vi "例程03-For、while循环、条件结构、事件结构.vi"() -> ()   [LabVIEW 2018]
panel:
  out "数值":dbl
  in  "事件结构测试":bool
  out "while次数 2":i32
  out "布尔":bool
  out "while次数":i32
  out "波形图表 2":dbl(graph)
  out "for次数":i32
  out "波形图表":dbl(graph)
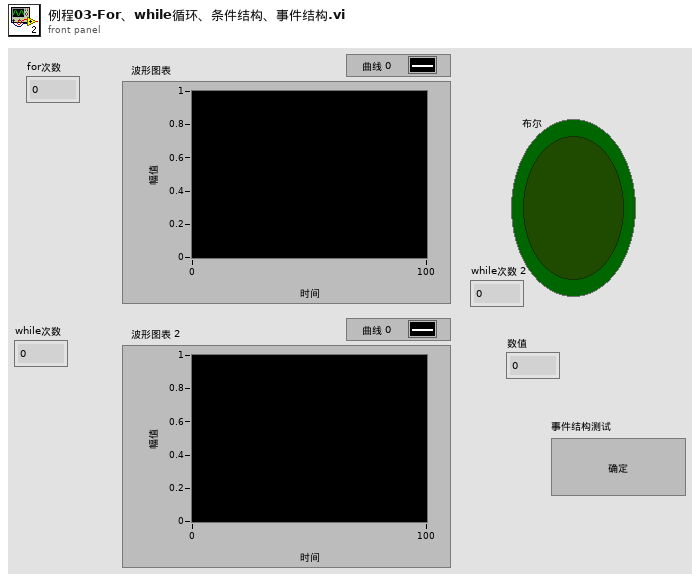
[diagram p1: front panel]
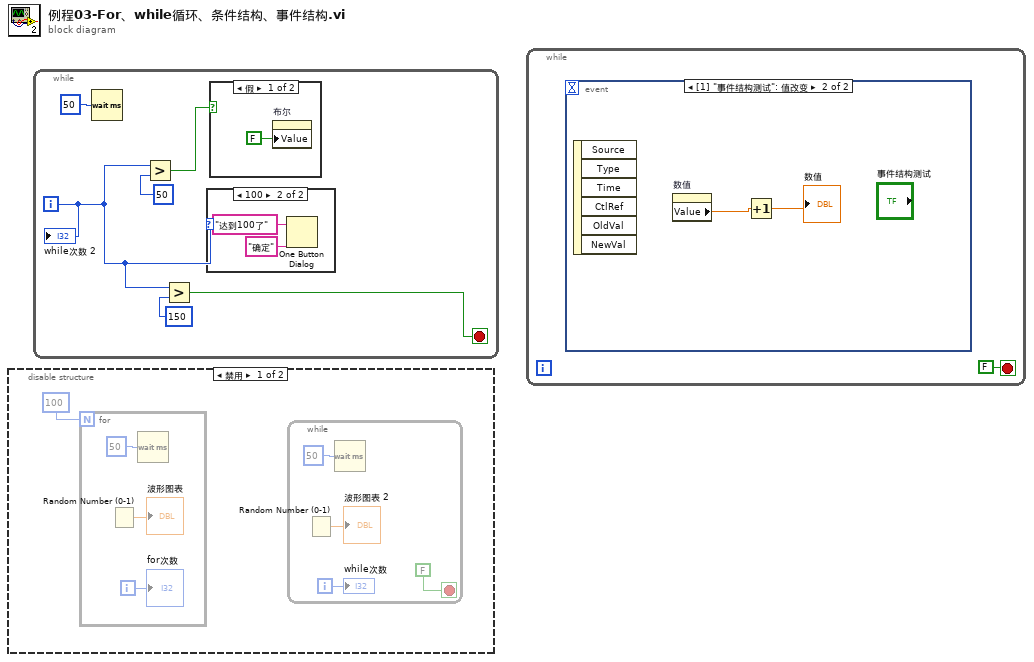
[diagram p0: block diagram]
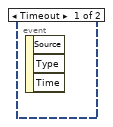
[diagram p2: hidden frame]
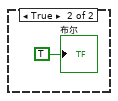
[diagram p5: hidden frame]
diagram:
  n1 = disable-structure shown="禁用" {
    frame Disabled {
      n2 = for {
        N: 100 -> [_]
        i -> [w6]
        n3 = Random Number (0-1)() -> (number: 0 to 1=→"波形图表":dbl)
        n4 = Wait (ms)(milliseconds to wait=u32 50 ("等待时间（毫秒）")) -> ()  [unwired: 1 out]
        "for次数" <- w6
      }
      n5 = while {
        i -> [w2]
        stop <- FALSE stop-if-true
        n6 = Random Number (0-1)() -> (number: 0 to 1=→"波形图表 2":dbl)
        n7 = Wait (ms)(milliseconds to wait=u32 50 ("等待时间（毫秒）")) -> ()  [unwired: 1 out]
        "while次数" <- w2
      }
    }
    frame Enabled {
    }
  }
  n8 = while {
    i -> [w10]
    stop <- w9 stop-if-true
    n9 = Wait (ms)(milliseconds to wait=u32 50 ("等待时间（毫秒）")) -> ()  [unwired: 1 out]
    n10 = Greater?(x=w10, y=50) -> (0:w12:bool)
    n11 = Greater?(x=w10, y=150) -> (0:w9:bool)
    n12 = case shown="100" w10 {
      frame 0, Default {
      }
      frame 100 {
        n13 = One Button Dialog(message="达到100了" ("消息"), button name ("OK")="确定" ("按钮名称（“确定”）")) -> ()  [unwired: 1 out]
      }
    }
    n14 = case shown="假" w12 {
      frame False {
        n15 = property on="布尔" class="Bool (严格)"("Value"=FALSE) -> ()  [unwired: 2 in, 2 out]
      }
      frame True {
        "布尔" <- TRUE
      }
    }
    "while次数 2" <- w10
  }
  n16 = while {
    stop <- FALSE stop-if-true
    n17 = event shown="[1] \"事件结构测试\": 值改变" {
      selector: _ -> [_ _]
      dyn-events: _ -> [_ _]
      timeout: _ -> [_ _]
      event Timeout {
        n18 = event-data() -> ()  [unwired: 1 in, 3 out]
      }
      event "事件结构测试": Value Change {
        n19 = event-data() -> ()  [unwired: 1 in, 6 out]
        n20 = property on="数值" class="DigNum (严格)"() -> ("Value"=w21:dbl)  [unwired: 2 in, 2 out]
        n21 = Increment(x=w21) -> (x+1=→"数值":dbl)
      }
    }
  }
